vi "Get PressureDisplay Setup.vi"(8 "error in (no error)":errorcluster, 11 "VacuumLines Configuration in":refnum<class "VacuumLines Configuration.lvclass">) -> (0 "error out":errorcluster, 2 "PressureDisplay Setup":T1[](array[typedef]) {"Threshold" format="%#.1e"}, 3 "VacuumLines Configuration out":refnum<class "VacuumLines Configuration.lvclass">)   [LabVIEW 2016, in "Hardware.lvlib" / "VacuumLine.lvlib" / "VacuumLines Configuration.lvclass"]
uses:
  <userlib>/Common Components/Hardware/Abstract System/VacuumLine/VacuumLines Configuration/VacuumLines Configuration.lvclass
  <userlib>/Common Components/Hardware/Abstract System/VacuumLine/VacuumLines/Gauge Param.ctl
  <userlib>/Common Components/Hardware/Abstract System/VacuumLine/VacuumLines Configuration/VacuumLines Configuration.lvclass/VacuumLines Configuration.ctl
  <userlib>/Common Components/Hardware/Abstract System/VacuumLine/VacuumLines/VacuumLines.lvclass/VacuumLines.ctl
  <userlib>/Common Components/Hardware/Abstract System/VacuumLine/VacuumLines/VacuumLines.lvclass
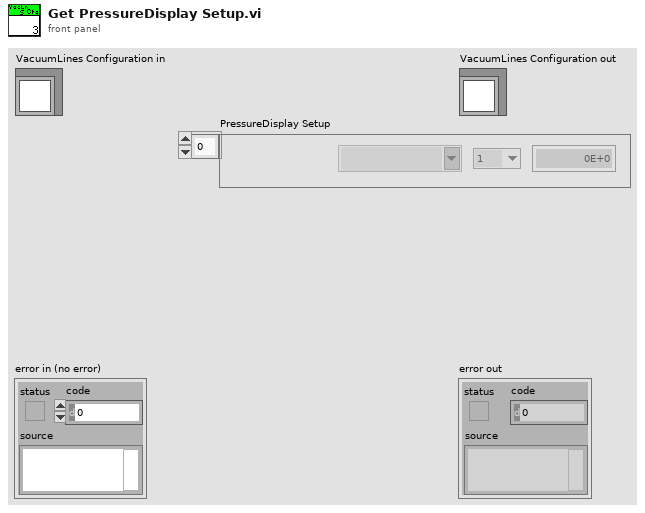
[diagram p1: front panel]
types:
  T1 = typedef "Hardware.lvlib/VacuumLine.lvlib/VacuumLines.lvclass/Gauge Param.ctl" = cluster{"label":string, "Gauge Controller":string, "Channel":enum16{"1", "2", "3", "4", "5", "6", "7", "8"}, "Threshold":dbl}
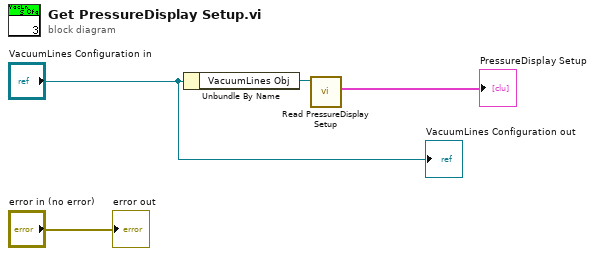
[diagram p0: block diagram]
diagram:
  n1 = Unbundle By Name("VacuumLines Configuration in") -> ("VacuumLines Obj"=w3:refnum<class "VacuumLines.lvclass">)
  n2 = call <userlib>:"Read PressureDisplay Setup.vi"("VacuumLines in"=w3) -> ("PressureDisplay Setup"=→"PressureDisplay Setup":T1[])  [unwired: 9 in, 1 out]
  "error out" <- "error in (no error)"
  "VacuumLines Configuration out" <- "VacuumLines Configuration in"
